vi "AddEISGalvanostatic.vi"(0 "deviceName":string, 1 "quietTimeSamplingInterval":sgl=1.0, 2 "endFreq":sgl=100.0, 3 "biasCurrent":sgl, 5 "channel":u8, 7 "repeats":u16=1, 9 "quietTime":sgl, 10 "minimumCycles":u32=2, 11 "error in (no error)":errorcluster, 12 "startFreq":sgl=1000.0, 13 "stepsPerDecade":sgl=10.0, 14 "amplitude":sgl) -> (15 "error out":errorcluster)   [LabVIEW 2018]
doc: "EXPORT void AisAddEISGalvanostatic(const char* deviceName, uint8_t channel, uint16_t repeats, float quietTime, float quietTimeSamplingInterval, float startFreq, float endFreq, float stepsPerDecade, float biasCurrent, float amplitude, unsigned int minimumCycles);"
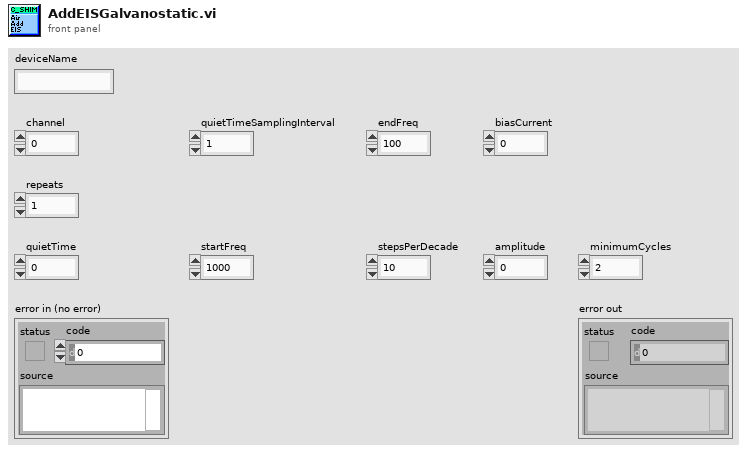
[diagram p1: front panel]
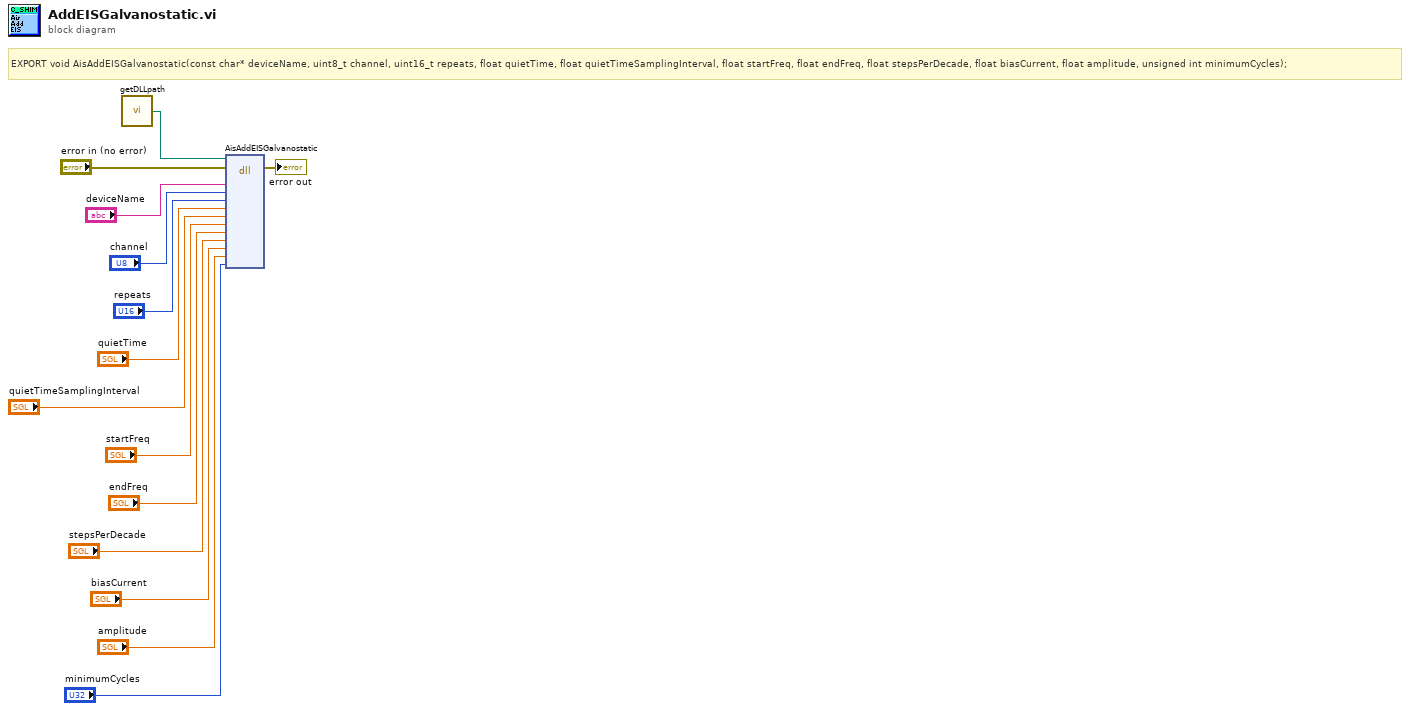
[diagram p0: block diagram]
diagram:
  # "EXPORT void AisAddEISGalvanostatic(const char* deviceName, uint8_t channel, uint16_t repeats, float quietTime, float quietTimeSamplingInterval, float startFreq, float endFreq, float stepsPerDecade, float biasCurrent, float amplitude, unsigned int minimumCycles);"
  n1 = call "getDLLpath.vi"() -> ("DLL_Path"=w1:path)
  n2 = dll-call lib="?" fn="AisAddEISGalvanostatic"(path in=w1, error in="error in (no error)", "deviceName"="deviceName", "channel"="channel", "repeats"="repeats", "quietTime"="quietTime", "quietTimeSamplingInterval"="quietTimeSamplingInterval", "startFreq"="startFreq", "endFreq"="endFreq", "stepsPerDecade"="stepsPerDecade", "biasCurrent"="biasCurrent", "amplitude"="amplitude", "minimumCycles"="minimumCycles") -> (error out=→"error out":errorcluster)  [unwired: 13 in, 1 out]
